vi "System Integrity Tool.vi"() -> ()   [LabVIEW 2010]
uses:
  SIT_Data.ctl
  Re-use Library/VIE.Module.Queued Message Handler.enqueue.State.PolyChild.QueuedMessageHandler.vi
  Re-use Library/VIE.Module.Queued Message Handler.[enqueue].State.PolyChild.QueuedMessageHandler.vi
  <vilib>/Utility/config.llb/Read Key (String).vi
  Re-use Library/Remove Duplicates from 1D Array (Path)__ogtk.vi
  Re-use Library/VIE.Module.Queued Message Handler.QueuedMessageHandler.dqGOOPClass.lvlib
  <vilib>/Utility/config.llb/NI_LVConfig.lvlib
panel:
  out "Error Out":errorcluster
  in  "Exit":bool
  in  "Add Package Integrity File":bool
  in  "Delete Package Integrity File":bool
  in  "Package Integrity Files":i32(listbox)
  in  "System Integrity File Path":path
  in  "Save System Integrity File":bool
  in  "User Name":string
  in  "Purpose":string
  in  "Package Revision":string
  in  "Package ID":string
  in  "Package Integrity File Path":path
  in  "Undo":bool
  in  "Save Package Integrity File":bool
  in  "Remove Selected Files":bool
  in  "Add VI Hierarchy":bool
  in  "Recursive":bool
  in  "Add Directory":bool
  in  "Add File":bool
  out "Selection Log":string
  in  "File List":i32[](listbox)
  in  "error in (no error)":errorcluster
  out "error out":errorcluster
  out "CVT (out)":T1
  # "Use the CVT as a data bus for data that is\nto be accesed outside of the VI.  It can be\nused for data passed around  inside the state\nmachine too, and all local data can be selectively\npurged from the CVT in the \"system.Exit\" state."
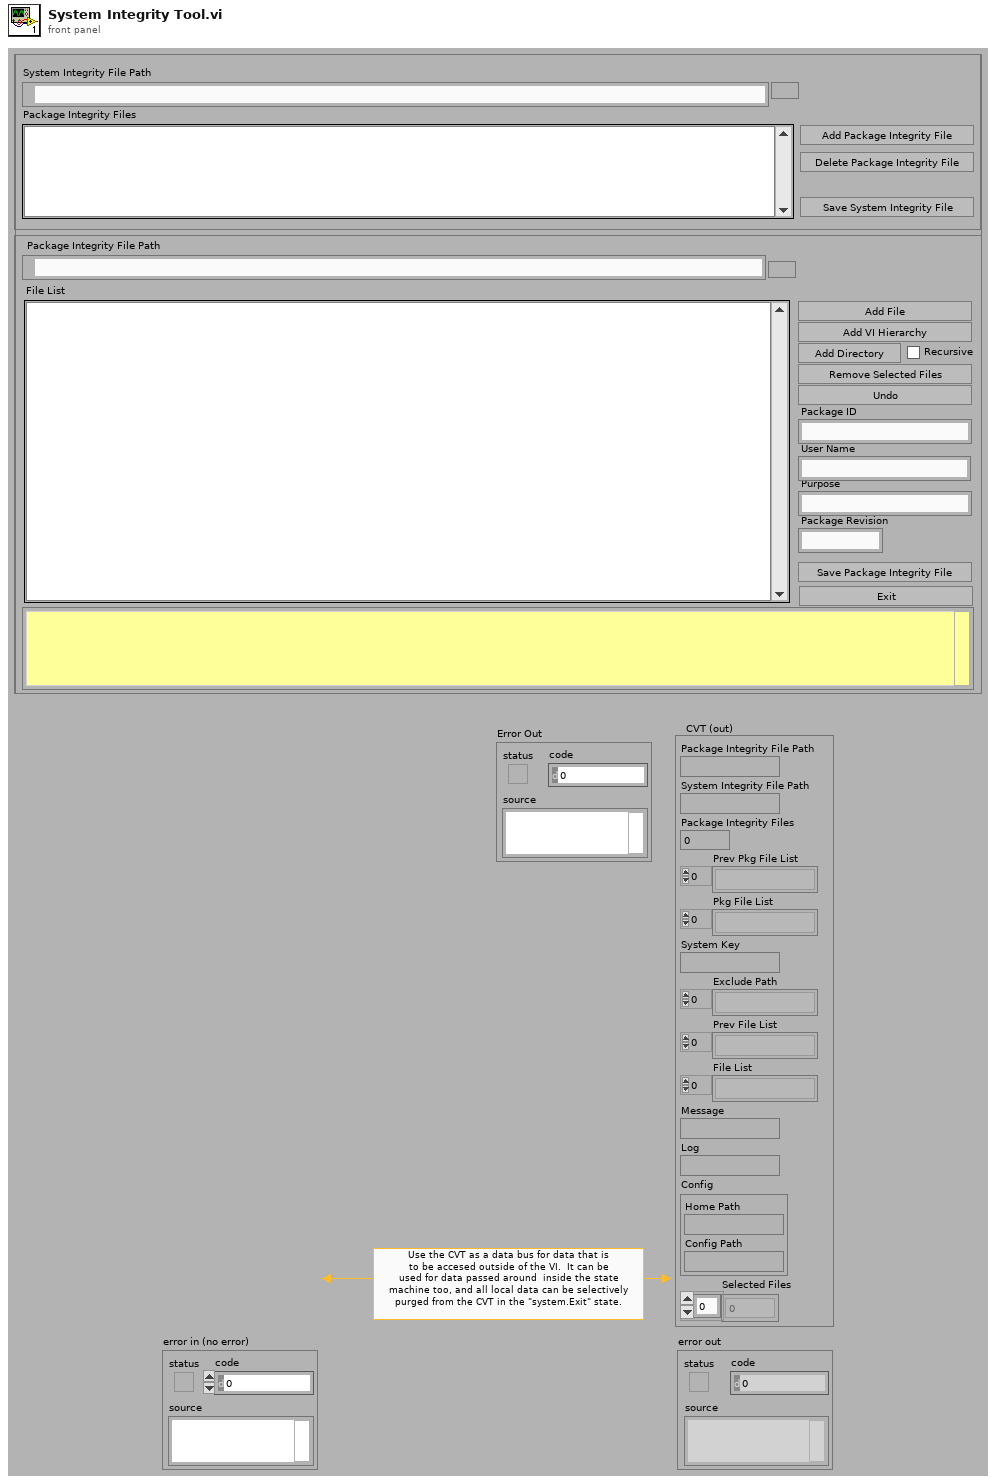
[diagram p1: front panel]
types:
  T1 = typedef "SIT_Data.ctl" = cluster{"Package Integrity File Path":path, "System Integrity File Path":path, "Package Integrity Files":i32, "Prev Pkg File List":path[], "Pkg File List":path[], "System Key":string, "Exclude Path":path[], "Prev File List":path[], "File List":path[], "Message":string, "Log":string, "Config":cluster{"Home Path":path, "Config Path":path}, "Selected Files":i32[]}
  T2 = typedef "VIE.Module.Queued Message Handler.QueuedMessageHandler.dqGOOPClass.lvlib/VIE.Module.Queued Message Handler.dqClass_ObjectReference.ctl" = refnum<k1>
  T3 = typedef "NI_LVConfig.lvlib/Config Data RefNum.ctl" = refnum<k1>
  T4 = enum32{"existing file", "new file", "new or existing file", "existing dir", "new dir", "new or existing dir", "existing file (use LLBs)", "new file (use LLBs)", "new or existing file (use LLBs)", "new or existing file or directory (use LLBs)", "existing dir (use LLBs)", "new dir (use LLBs)", "new or existing dir (use LLBs)", "existing file or dir", "new file or dir", "new or existing file or dir", "existing file or dir (use LLBs)", "new file or dir (use LLBs)"}
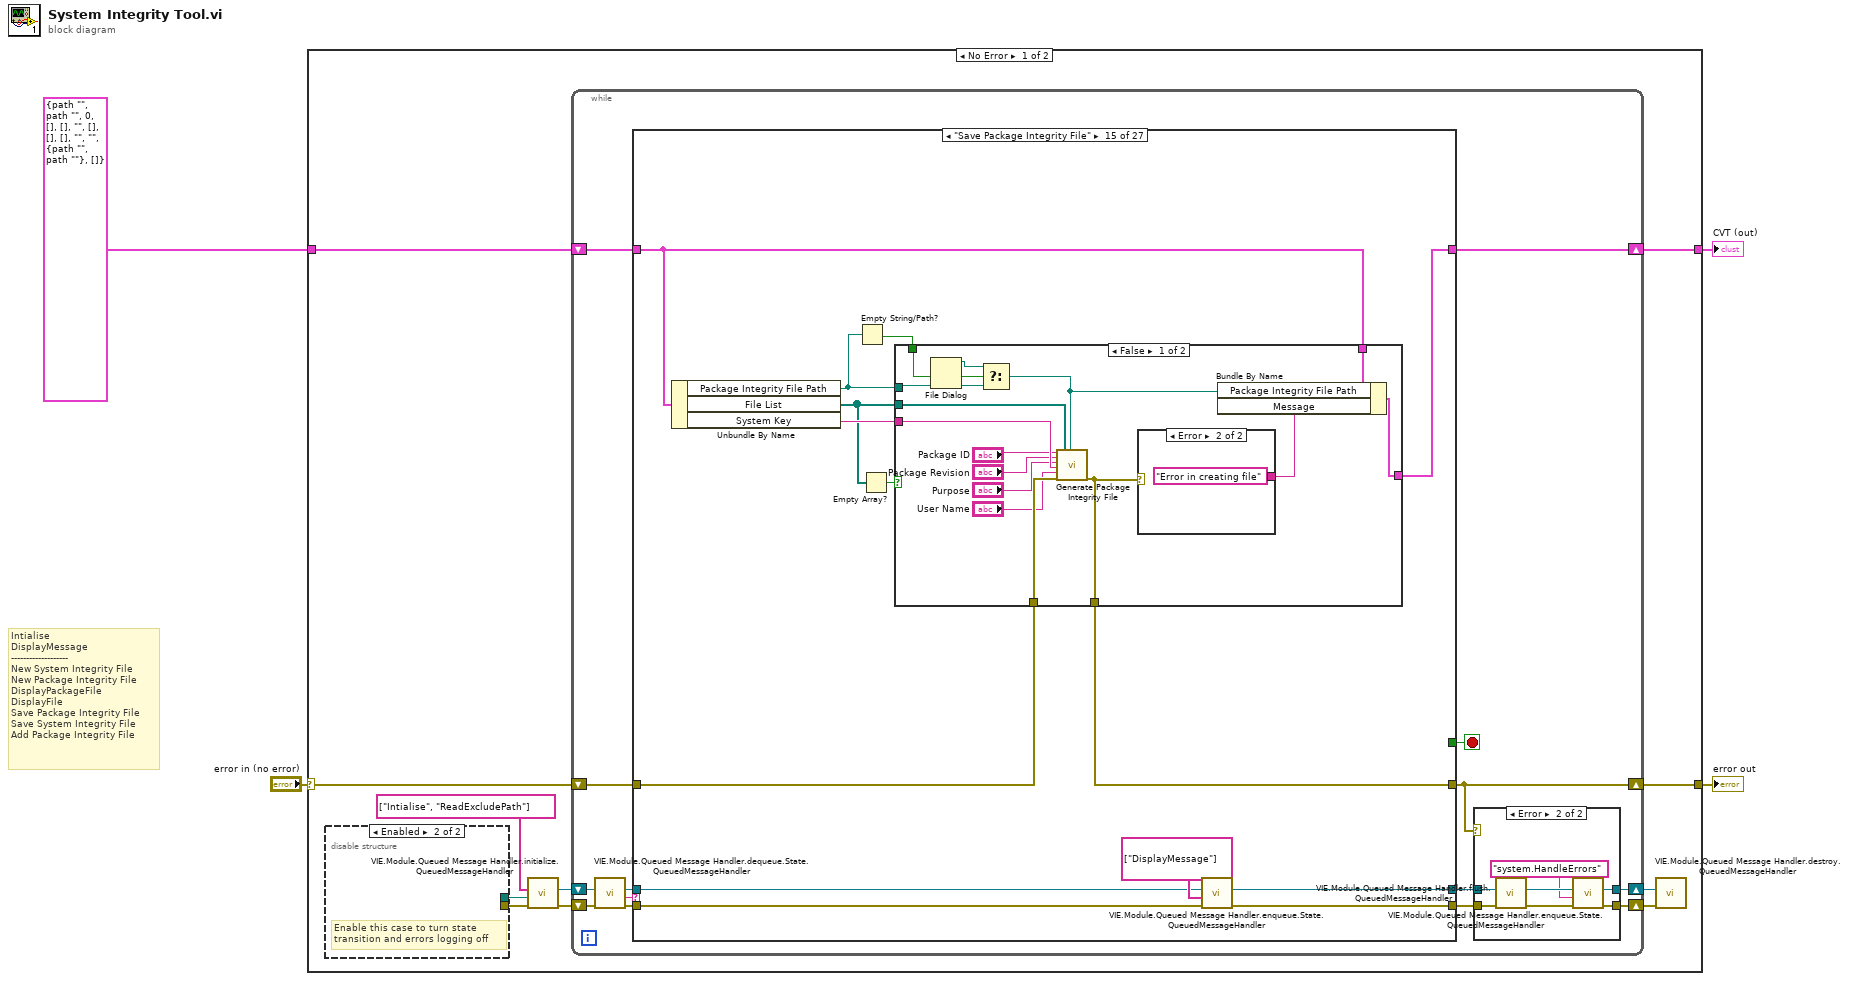
[diagram p0: block diagram]
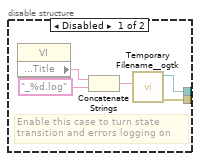
[diagram p2: hidden frame]
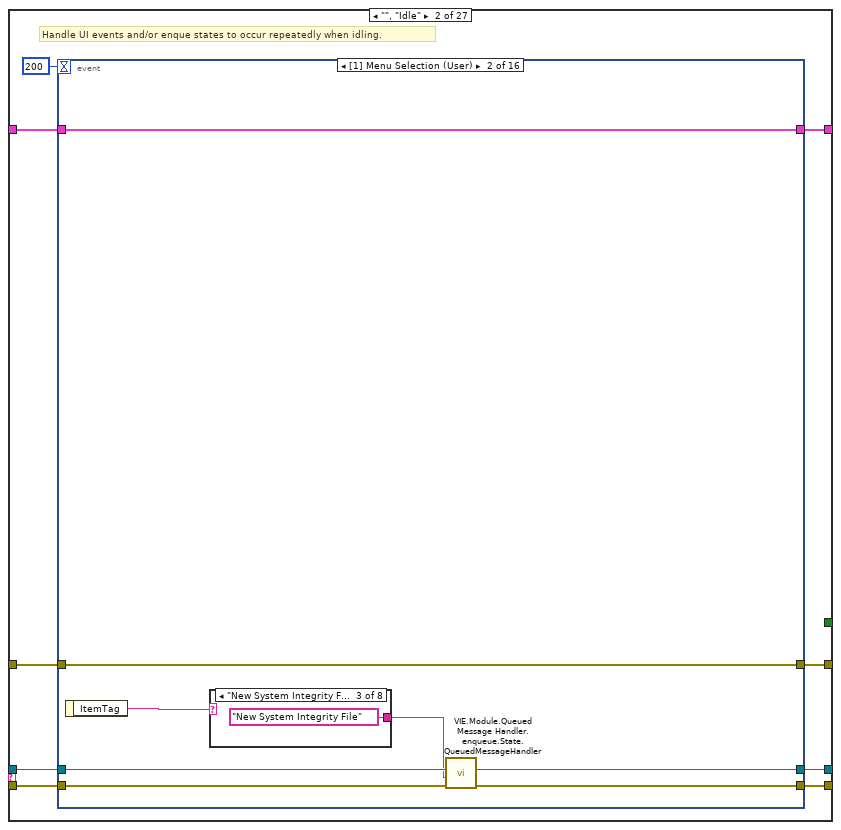
[diagram p5: hidden frame]
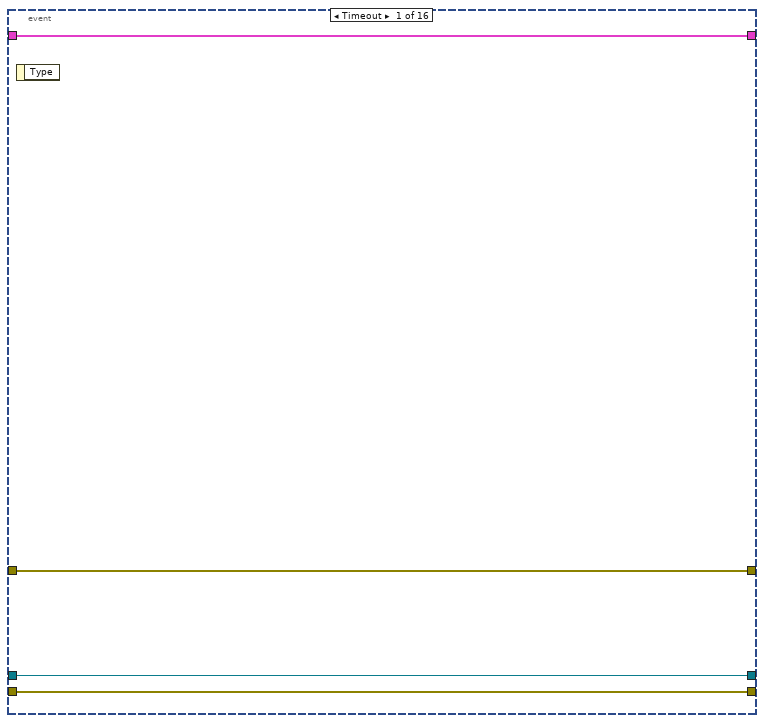
[diagram p6: hidden frame]
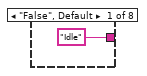
[diagram p7: hidden frame]
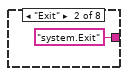
[diagram p8: hidden frame]
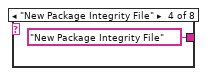
[diagram p9: hidden frame]
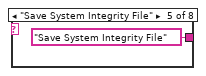
[diagram p10: hidden frame]
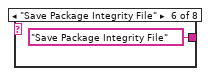
[diagram p11: hidden frame]
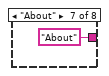
[diagram p12: hidden frame]
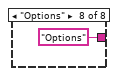
[diagram p13: hidden frame]
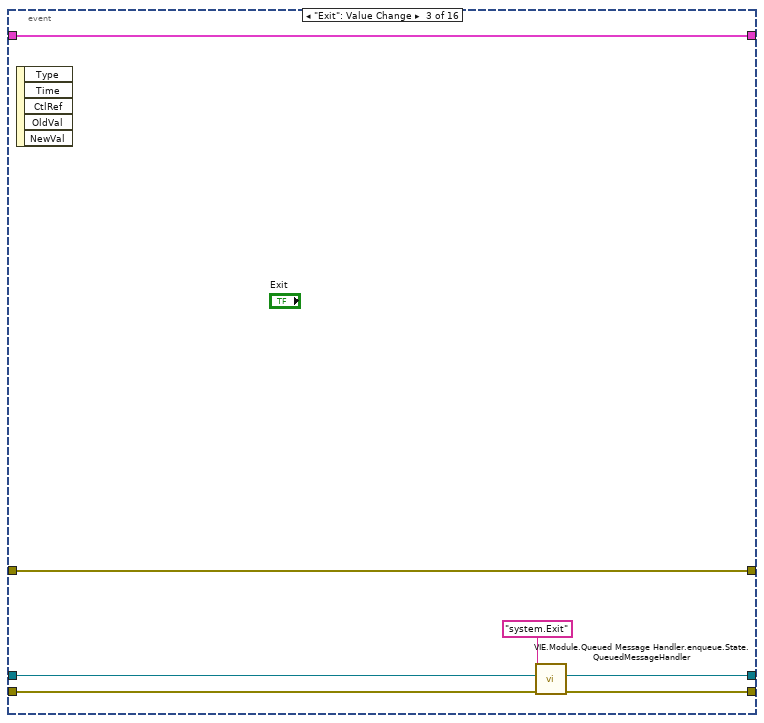
[diagram p14: hidden frame]
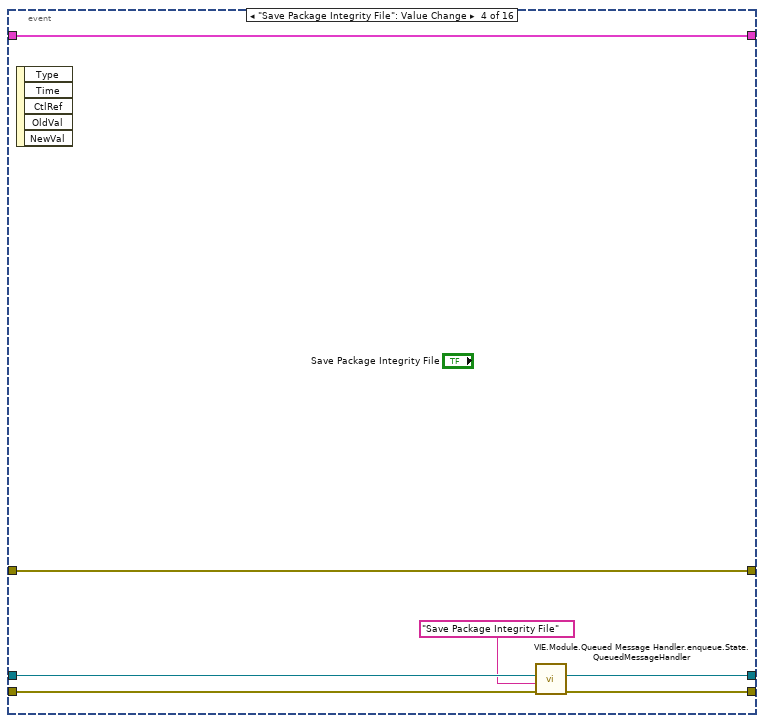
[diagram p15: hidden frame]
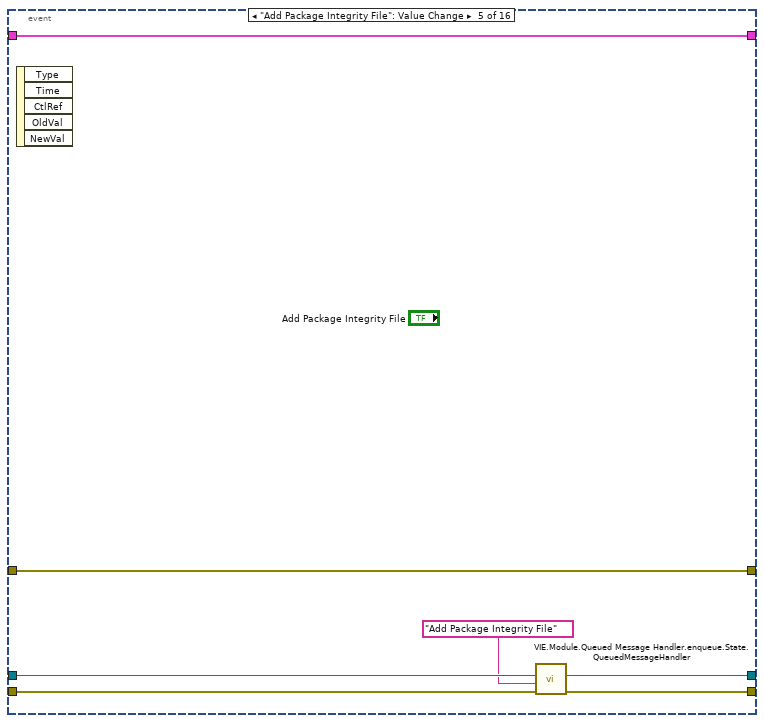
[diagram p16: hidden frame]
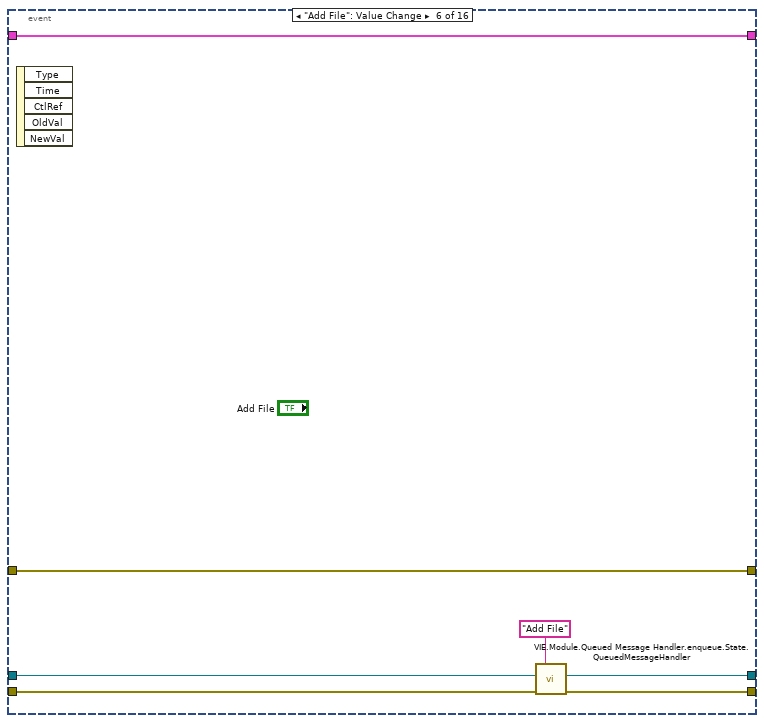
[diagram p17: hidden frame]
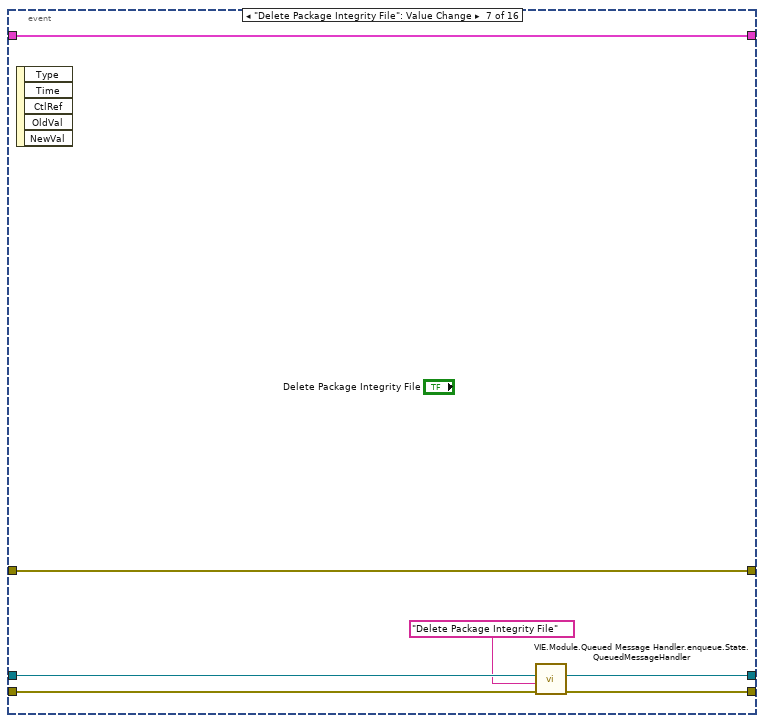
[diagram p18: hidden frame]
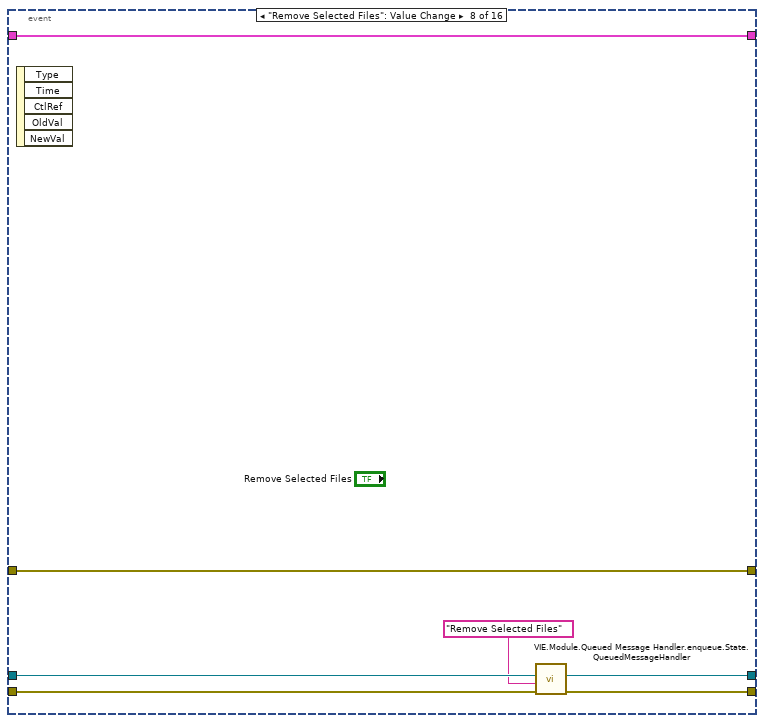
[diagram p19: hidden frame]
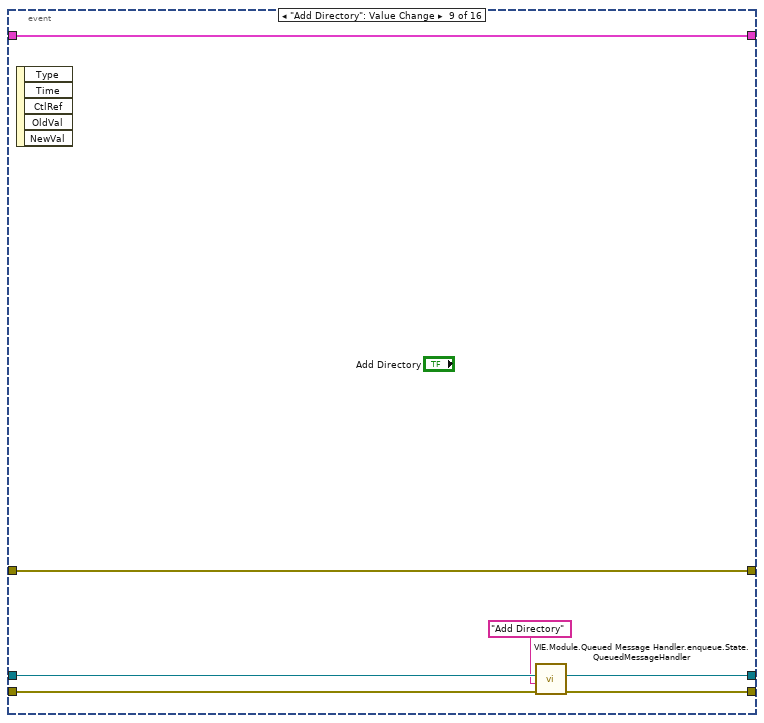
[diagram p20: hidden frame]
diagram:
  # "Intialise\nDisplayMessage\n-------------------\nNew System Integrity File\nNew Package Integrity File\nDisplayPackageFile\nDisplayFile\nSave Package Integrity File\nSave System Integrity File\nAdd Package Integrity File"
  n1 = case shown="No Error" "error in (no error)" {
    selector: "error in (no error)" -> [w8 w719]
    tunnel: [w7 w719] -> w2
    tunnel: T1 {"Package Integrity File Path"=path "", "System Integrity File Path"=path "", "Package Integrity Files"=0, "Prev Pkg File List"=[], "Pkg File List"=[], "System Key"="", "Exclude Path"=[], "Prev File List"=[], "File List"=[], "Message"="", "Log"="", "Config"={"Home Path"=path "", "Config Path"=path ""}, "Selected Files"=[]} ("CVT (in)") -> [w5 w718]
    tunnel: [w9 w718] -> w4
    frame No Error {
      n2 = disable-structure shown="Enabled" {
        disable-tunnel: [w17 _] -> w11
        disable-tunnel: [w16 _] -> w10
        frame Disabled {
          # "Enable this case to turn state\ntransition and errors logging on"
          n3 = property class="VI"() -> ("Front Panel.Title"=w18:string)  [unwired: 2 in, 2 out]
          n4 = Concatenate Strings(w18, "_%d.log" ("string")) -> (w20:string)
          n5 = call <userlib>:"Temporary Filename__ogtk.vi"("pattern (lvtemp%d.tmp)"=w20) -> ("error out"=w17:errorcluster, "file in tmp dir"=w16:path)  [unwired: 5 in]
        }
        frame Enabled {
          # "Enable this case to turn state\ntransition and errors logging off"
        }
      }
      n6 = call "VIE.Module.Queued Message Handler.initialize.QueuedMessageHandler.vi"("error in (no error)"=w11, "State Queue Log FilePath (\"\" = Do Not Log)"=w10, "Initial State Queue (empty)"=string[] ["Intialise", "ReadExcludePath"] ("Initial State Queue")) -> ("error out"=w15:errorcluster, "QueuedMessageHandler.dqGOOPClass (out)"=w12:T2)  [unwired: 7 in]
      n7 = while {
        shift-right: [w23] -> w14
        shift-left: w15 -> [w31]
        shift-right: [w28] -> w9
        shift-left: w5 -> [w29]
        shift-right: [w26] -> w7
        shift-left: w8 -> [w27]
        shift-right: [w22] -> w13
        shift-left: w12 -> [w34]
        stop <- w21 stop-if-true
        n8 = call "VIE.Module.Queued Message Handler.dequeue.State.QueuedMessageHandler.vi"("error in (no error)"=w31, "QueuedMessageHandler.dqGOOPClass (in)"=w34) -> ("error out"=w32:errorcluster, "State Dequeued"=w30:string, "QueuedMessageHandler.dqGOOPClass (out)"=w33:T2)  [unwired: 7 in]
        n9 = case shown="\"Save Package Integrity File\"" w30 {
          selector: w30 -> [_ _ _ _ _ _ _ _ _ _ _ _ _ _ _ _ _ _ _ _ _ _ _ _ w679 _ _]
          tunnel: w32 -> [w44 w54 w192 w199 w220 w225 w250 w256 w262 w278 w293 w334 w345 w373 w406 w442 w459 w492 w522 w555 w610 w625 w635 w673 w678 w696 w714]
          tunnel: [w44 w49 w189 w199 w220 w224 w248 w255 w262 w276 w291 w332 w344 w372 w405 w441 w458 w491 w521 w554 w609 w624 w634 w673 w678 w687 w714] -> w25
          tunnel: w33 -> [w45 w53 w191 w200 w221 w223 w251 w254 w263 w279 w294 w335 w343 w371 w404 w440 w457 w490 w520 w553 w608 w623 w633 w674 w677 w697 w715]
          tunnel: [w45 w50 w190 w200 w221 w222 w249 w253 w263 w277 w292 w333 w342 w370 w403 w439 w456 w489 w519 w552 w607 w622 w632 w674 w677 w688 w715] -> w24
          tunnel: w29 -> [w47 w56 w196 w202 w211 w234 w252 w259 w265 w272 w285 w324 w351 w376 w401 w433 w451 w484 w516 w549 w606 w621 w639 w676 w686 w700 w713]
          tunnel: [w47 w52 w195 w206 w210 w233 w252 w259 w265 w271 w289 w323 w350 w375 w400 w432 w450 w483 w515 w548 w605 w620 w638 w676 w686 w700 w713] -> w28
          tunnel: w27 -> [w46 w55 w197 w201 w219 w235 w246 w260 w264 w274 w287 w330 w356 w384 w399 _ w449 w482 w514 w547 w604 w619 w654 w675 w681 w698 w716]
          tunnel: [w46 w51 w183 w203 w219 w235 w246 w260 w264 w274 w286 w330 w356 w384 w398 w429 w448 w481 w513 w546 w604 w619 w654 w675 w680 w691 w716] -> w26
          tunnel: [_ _ _ _ _ _ _ _ _ _ _ _ _ _ _ _ _ _ _ _ _ _ _ _ _ _ TRUE] -> w21
          frame "---- Custom States --------------------------" {
            # "Do not put any code in here - this is a case divider, and is not a valid state, so any code here will not be executed."
          }
          frame "", "Idle" {
            # "Handle UI events and/or enque states to occur repeatedly when idling."
            n10 = event shown="[1] Menu Selection (User)" {
              selector: _ -> [_ _ _ _ _ _ _ _ _ _ _ _ _ _ _ _]
              dyn-events: _ -> [_ _ _ _ _ _ _ _ _ _ _ _ _ _ _ _]
              timeout: 200 -> [_ _ _ _ _ _ _ _ _ _ _ _ _ _ _ _]
              tunnel: w56 -> [w60 w68 w83 w90 w97 w104 w111 w118 w125 w132 w139 w146 w149 w159 w168 w179]
              tunnel: w55 -> [w57 w67 w82 w89 w96 w103 w110 w117 w124 w131 w138 w145 w155 w166 w175 w181]
              tunnel: w54 -> [w58 w66 w81 w88 w95 w102 w109 w116 w123 w130 w137 w144 w154 w165 w174 w176]
              tunnel: w53 -> [w59 w64 w79 w86 w93 w100 w107 w114 w121 w128 w135 w142 w152 w163 w172 w177]
              tunnel: [w60 w68 w83 w90 w97 w104 w111 w118 w125 w132 w139 w146 w148 w160 w169 w180] -> w52
              tunnel: [w57 w67 w82 w89 w96 w103 w110 w117 w124 w131 w138 w145 w155 w166 w175 w181] -> w51
              tunnel: [w59 w63 w78 w85 w92 w99 w106 w113 w120 w127 w134 w141 w151 w162 w171 w177] -> w50
              tunnel: [w58 w65 w80 w87 w94 w101 w108 w115 w122 w129 w136 w143 w153 w164 w173 w176] -> w49
              event Timeout {
                n11 = event-data() -> ()  [unwired: 1 in, 1 out]
              }
              event Menu Selection (User) {
                n12 = event-data() -> ("ItemTag"=w62:string)  [unwired: 1 in]
                n13 = case shown="\"New System Integrity File\"" w62 {
                  tunnel: ["Idle" ("ItemTag") "system.Exit" ("ItemTag") "New System Integrity File" ("ItemTag") "New Package Integrity File" ("ItemTag") "Save System Integrity File" ("ItemTag") "Save Package Integrity File" ("ItemTag") "About" ("ItemTag") "Options" ("ItemTag")] -> w61
                  frame "False", Default {
                  }
                  frame "Exit" {
                  }
                  frame "New System Integrity File" {
                  }
                  frame "New Package Integrity File" {
                  }
                  frame "Save System Integrity File" {
                  }
                  frame "Save Package Integrity File" {
                  }
                  frame "About" {
                  }
                  frame "Options" {
                  }
                }
                n14 = call-poly "VIE.Module.Queued Message Handler.enqueue.State.QueuedMessageHandler.vi"("error in (no error)"=w66, "State to Enqueue"=w61, "QueuedMessageHandler.dqGOOPClass (in)"=w64) -> ("error out"=w65:errorcluster, "QueuedMessageHandler.dqGOOPClass (out)"=w63:T2)  [unwired: 7 in]
              }
              event "Exit": Value Change {
                n15 = event-data() -> ()  [unwired: 1 in, 5 out]
                n16 = call-poly "VIE.Module.Queued Message Handler.enqueue.State.QueuedMessageHandler.vi"("error in (no error)"=w81, "State to Enqueue"="system.Exit", "QueuedMessageHandler.dqGOOPClass (in)"=w79) -> ("error out"=w80:errorcluster, "QueuedMessageHandler.dqGOOPClass (out)"=w78:T2)  [unwired: 7 in]
              }
              event "Save Package Integrity File": Value Change {
                n17 = event-data() -> ()  [unwired: 1 in, 5 out]
                n18 = call-poly "VIE.Module.Queued Message Handler.enqueue.State.QueuedMessageHandler.vi"("error in (no error)"=w88, "State to Enqueue"="Save Package Integrity File", "QueuedMessageHandler.dqGOOPClass (in)"=w86) -> ("error out"=w87:errorcluster, "QueuedMessageHandler.dqGOOPClass (out)"=w85:T2)  [unwired: 7 in]
              }
              event "Add Package Integrity File": Value Change {
                n19 = event-data() -> ()  [unwired: 1 in, 5 out]
                n20 = call-poly "VIE.Module.Queued Message Handler.enqueue.State.QueuedMessageHandler.vi"("error in (no error)"=w95, "State to Enqueue"="Add Package Integrity File", "QueuedMessageHandler.dqGOOPClass (in)"=w93) -> ("error out"=w94:errorcluster, "QueuedMessageHandler.dqGOOPClass (out)"=w92:T2)  [unwired: 7 in]
              }
              event "Add File": Value Change {
                n21 = event-data() -> ()  [unwired: 1 in, 5 out]
                n22 = call-poly "VIE.Module.Queued Message Handler.enqueue.State.QueuedMessageHandler.vi"("error in (no error)"=w102, "State to Enqueue"="Add File", "QueuedMessageHandler.dqGOOPClass (in)"=w100) -> ("error out"=w101:errorcluster, "QueuedMessageHandler.dqGOOPClass (out)"=w99:T2)  [unwired: 7 in]
              }
              event "Delete Package Integrity File": Value Change {
                n23 = event-data() -> ()  [unwired: 1 in, 5 out]
                n24 = call-poly "VIE.Module.Queued Message Handler.enqueue.State.QueuedMessageHandler.vi"("error in (no error)"=w109, "State to Enqueue"="Delete Package Integrity File", "QueuedMessageHandler.dqGOOPClass (in)"=w107) -> ("error out"=w108:errorcluster, "QueuedMessageHandler.dqGOOPClass (out)"=w106:T2)  [unwired: 7 in]
              }
              event "Remove Selected Files": Value Change {
                n25 = event-data() -> ()  [unwired: 1 in, 5 out]
                n26 = call-poly "VIE.Module.Queued Message Handler.enqueue.State.QueuedMessageHandler.vi"("error in (no error)"=w116, "State to Enqueue"="Remove Selected Files", "QueuedMessageHandler.dqGOOPClass (in)"=w114) -> ("error out"=w115:errorcluster, "QueuedMessageHandler.dqGOOPClass (out)"=w113:T2)  [unwired: 7 in]
              }
              event "Add Directory": Value Change {
                n27 = event-data() -> ()  [unwired: 1 in, 5 out]
                n28 = call-poly "VIE.Module.Queued Message Handler.enqueue.State.QueuedMessageHandler.vi"("error in (no error)"=w123, "State to Enqueue"="Add Directory", "QueuedMessageHandler.dqGOOPClass (in)"=w121) -> ("error out"=w122:errorcluster, "QueuedMessageHandler.dqGOOPClass (out)"=w120:T2)  [unwired: 7 in]
              }
              event "Add VI Hierarchy": Value Change {
                n29 = event-data() -> ()  [unwired: 1 in, 5 out]
                n30 = call-poly "VIE.Module.Queued Message Handler.enqueue.State.QueuedMessageHandler.vi"("error in (no error)"=w130, "State to Enqueue"="Add VI Hierarchy", "QueuedMessageHandler.dqGOOPClass (in)"=w128) -> ("error out"=w129:errorcluster, "QueuedMessageHandler.dqGOOPClass (out)"=w127:T2)  [unwired: 7 in]
              }
              event "Undo": Value Change {
                n31 = event-data() -> ()  [unwired: 1 in, 5 out]
                n32 = call-poly "VIE.Module.Queued Message Handler.enqueue.State.QueuedMessageHandler.vi"("error in (no error)"=w137, "State to Enqueue"="Undo", "QueuedMessageHandler.dqGOOPClass (in)"=w135) -> ("error out"=w136:errorcluster, "QueuedMessageHandler.dqGOOPClass (out)"=w134:T2)  [unwired: 7 in]
              }
              event "Save System Integrity File": Value Change {
                n33 = event-data() -> ()  [unwired: 1 in, 5 out]
                n34 = call-poly "VIE.Module.Queued Message Handler.enqueue.State.QueuedMessageHandler.vi"("error in (no error)"=w144, "State to Enqueue"="Save System Integrity File", "QueuedMessageHandler.dqGOOPClass (in)"=w142) -> ("error out"=w143:errorcluster, "QueuedMessageHandler.dqGOOPClass (out)"=w141:T2)  [unwired: 7 in]
              }
              event "System Integrity File Path": Value Change {
                n35 = event-data() -> ("NewVal"=w147:path)  [unwired: 1 in]
                n36 = Bundle By Name(cluster=w149, "System Integrity File Path"=w147) -> (w148:T1)
                n37 = call-poly "VIE.Module.Queued Message Handler.enqueue.State.QueuedMessageHandler.vi"("error in (no error)"=w154, "State to Enqueue"="Load System Integrity File", "QueuedMessageHandler.dqGOOPClass (in)"=w152) -> ("error out"=w153:errorcluster, "QueuedMessageHandler.dqGOOPClass (out)"=w151:T2)  [unwired: 7 in]
              }
              event "Package Integrity Files": Value Change {
                n38 = event-data() -> ("NewVal"=w156:i32)  [unwired: 1 in]
                n39 = Unbundle By Name(w159) -> ("Pkg File List"=w158:path[])
                n40 = Index Array(array=w158, index=w156) -> (element=w157:path)
                n41 = local write "Package Integrity File Path"(w157) -> ()
                n42 = Bundle By Name(cluster=w159, "Package Integrity File Path"=w157, "Package Integrity Files"=w156) -> (w160:T1)
                n43 = call-poly "VIE.Module.Queued Message Handler.enqueue.State.QueuedMessageHandler.vi"("error in (no error)"=w165, "State to Enqueue"="Load Package Integrity File", "QueuedMessageHandler.dqGOOPClass (in)"=w163) -> ("error out"=w164:errorcluster, "QueuedMessageHandler.dqGOOPClass (out)"=w162:T2)  [unwired: 7 in]
              }
              event "Package Integrity File Path": Value Change {
                n44 = event-data() -> ()  [unwired: 1 in, 1 out]
                n45 = Bundle By Name(cluster=w168, "Package Integrity File Path"="Package Integrity File Path") -> (w169:T1)
                n46 = call-poly "VIE.Module.Queued Message Handler.enqueue.State.QueuedMessageHandler.vi"("error in (no error)"=w174, "State to Enqueue"="Load Package Integrity File", "QueuedMessageHandler.dqGOOPClass (in)"=w172) -> ("error out"=w173:errorcluster, "QueuedMessageHandler.dqGOOPClass (out)"=w171:T2)  [unwired: 7 in]
              }
              event "File List": Value Change {
                n47 = event-data() -> ("NewVal"=w178:i32[])  [unwired: 1 in]
                n48 = Bundle By Name(cluster=w179, "Selected Files"=w178) -> (w180:T1)
              }
            }
          }
          frame "Intialise" {
            w184 = path "" ("Package Integrity File Path")
            w185 = string[] [] ("Item Names")
            n49 = call "Fit VI window to Largest Dec__ogtk.vi"("error in (no error)"=w197) -> ("error out"=w183:errorcluster)  [unwired: 5 in, 1 out]
            n50 = Current VI's Path() -> (path=w187:path)
            n51 = Strip Path(path=w187) -> (stripped path=w186:path)  [unwired: 1 out]
            n52 = Build Path(base path=w186, name or relative path="System Integrity Tool setting.ini") -> (appended path=w182:path)
            n53 = local write "System Integrity File Path"(w184) -> ()
            n54 = local write "Package Integrity File Path"(w184) -> ()
            n55 = Bundle By Name(cluster=w196, "Message"="Welcome to the Package Integrity File Generation Utility, brought to you by VI Engineering, Inc." ("queue element"), "Config.Home Path"=w186, "Config.Config Path"=w182) -> (w195:T1)
            n56 = property on="Package Integrity Files" class="LstBox (strict)"("Item Names"=w185) -> ()  [unwired: 2 in, 2 out]
            n57 = property on="File List" class="LstBox (strict)"("Item Names"=w185) -> ()  [unwired: 2 in, 2 out]
            n58 = call-poly "VIE.Module.Queued Message Handler.enqueue.State.QueuedMessageHandler.vi"("error in (no error)"=w192, "State to Enqueue"="DisplayMessage", "QueuedMessageHandler.dqGOOPClass (in)"=w191) -> ("error out"=w189:errorcluster, "QueuedMessageHandler.dqGOOPClass (out)"=w190:T2)  [unwired: 7 in]
          }
          frame "ReadExcludePath" {
            n59 = Unbundle By Name(w202) -> ("Config.Config Path"=w198:path)
            n60 = call "Read Write Exclude path.vi"("path In"=w198, "Error In"=w201) -> ("Key out"=w205:string, "Exclude Path Out"=w204:path[], "Error Out"=w203:errorcluster)  [unwired: 10 in, 1 out]
            n61 = Bundle By Name(cluster=w202, "System Key"=w205, "Exclude Path"=w204) -> (w206:T1)
          }
          frame "DisplayMessage" {
            n62 = Unbundle By Name(w211) -> ("Log"=w214:string, "Message"=w208:string)
            n63 = Empty String/Path?(string/path=w208) -> (empty?=w218:bool)
            n64 = Select(t="", s=w218, f="\r") -> (s? t:f=w216:string)
            n65 = Concatenate Strings(w214, w216, w208) -> (w213:string)
            n66 = call "SIT_Limit Display.vi"("Limit"=100 ("Number of Lines"), "Data In"=w213) -> ("Line Count"=w207:i32, "Data Out"=w209:string)  [unwired: 8 in]
            "Selection Log" <- w209
            n67 = property on="Selection Log" class="Str"("Text.Scroll Position"=w207) -> ()  [unwired: 2 in, 2 out]
            n68 = Bundle By Name(cluster=w211, "Log"=w209) -> (w210:T1)
          }
          frame "Undo" {
            n69 = Unbundle By Name(w234) -> ("Prev File List"=w228:path[], "File List"=w227:path[])
            n70 = Array Size(array=w228) -> (size(s)=w231:i32)
            n71 = Array Size(array=w227) -> (size(s)=w230:i32)
            n72 = Greater?(x=w231, y=w230) -> (0:w232:bool)
            n73 = case shown="True" w232 {
              tunnel: w231 -> [w238 w244]
              tunnel: w230 -> [w237 w243]
              tunnel: [w236 w241] -> w229
              frame False {
                n74 = Subtract(x=w237, y=w238) -> (x-y=w240:i32)
                n75 = Format Into String(format string="Undo: %d File(s) Removed from List" ("Format String"), w240) -> (resulting string=w236:string)  [unwired: 2 in, 1 out]
              }
              frame True {
                n76 = Subtract(x=w244, y=w243) -> (x-y=w242:i32)
                n77 = Format Into String(format string="Undo: %d File(s) Added Back to List" ("Format String"), w242) -> (resulting string=w241:string)  [unwired: 2 in, 1 out]
              }
            }
            n78 = call-poly "VIE.Module.Queued Message Handler.enqueue.State.QueuedMessageHandler.vi"("error in (no error)"=w225, "States to Enqueue"=string[] ["DisplayMessage", "DisplayFile"], "QueuedMessageHandler.dqGOOPClass (in)"=w223) -> ("error out"=w224:errorcluster, "QueuedMessageHandler.dqGOOPClass (out)"=w222:T2)  [unwired: 7 in]
            n79 = Bundle By Name(cluster=w234, "File List"=w228, "Prev File List"=w227, "Message"=w229) -> (w233:T1)
          }
          frame "custom.CleanUp" {
            n80 = call-poly "VIE.Module.Queued Message Handler.enqueue.State.QueuedMessageHandler.vi"("error in (no error)"=w250, "State to Enqueue"="system.Exit", "QueuedMessageHandler.dqGOOPClass (in)"=w251) -> ("error out"=w248:errorcluster, "QueuedMessageHandler.dqGOOPClass (out)"=w249:T2)  [unwired: 7 in]
          }
          frame "Options" {
            n81 = Unbundle By Name(w259) -> ("Config.Config Path"=w258:path)
            n82 = call "Exclude Path Options.vi"("Error In"=w260, "Path In"=w258) -> ()  [unwired: 9 in, 1 out]
            n83 = call-poly "VIE.Module.Queued Message Handler.enqueue.State.QueuedMessageHandler.vi"("error in (no error)"=w256, "State to Enqueue"="ReadExcludePath", "QueuedMessageHandler.dqGOOPClass (in)"=w254) -> ("error out"=w255:errorcluster, "QueuedMessageHandler.dqGOOPClass (out)"=w253:T2)  [unwired: 7 in]
          }
          frame "About" {
            n84 = One Button Dialog(message="Purpose of this tool is for System Integrity") -> ()  [unwired: 1 in, 1 out]
          }
          frame "Load Package Integrity File" {
            n85 = Unbundle By Name(w272) -> ("Package Integrity File Path"=w273:path)
            n86 = call "Load Package Config.vi"("Path"=w273) -> ("Path Out"=w270:path[], "Package ID"=w269:string, "Purpose"=w268:string, "Package Revision"=w267:string, "Error Out"=→"Error Out":errorcluster)  [unwired: 9 in, 1 out]
            n87 = local write "Purpose"(w268) -> ()
            n88 = local write "Package Revision"(w267) -> ()
            n89 = local write "Package ID"(w269) -> ()
            n90 = call-poly "VIE.Module.Queued Message Handler.enqueue.State.QueuedMessageHandler.vi"("error in (no error)"=w278, "State to Enqueue"="DisplayFile", "QueuedMessageHandler.dqGOOPClass (in)"=w279) -> ("error out"=w276:errorcluster, "QueuedMessageHandler.dqGOOPClass (out)"=w277:T2)  [unwired: 7 in]
            n91 = Bundle By Name(cluster=w272, "Prev File List"=w270, "File List"=w270) -> (w271:T1)
          }
          frame "Load System Integrity File" {
            n92 = Unbundle By Name(w285) -> ("System Integrity File Path"=w284:path)
            n93 = call <vilib>:"Open Config Data.vi"("error in (no error)"=w287, "create file if necessary (T)"=FALSE, "configuration file path"=w284) -> ("error out"=w280:errorcluster, "refnum"=w288:T3)  [unwired: 6 in, 1 out]
            n94 = case shown="No Error" w280 {
              selector: w280 -> [w295 _]
              tunnel: w288 -> [w300 _]
              tunnel: [w299 _] -> w286
              tunnel: [w298 _] -> w283
              frame No Error {
                w306 = "Package Integrity Files" ("section")
                n95 = call <vilib>:"Get Key Names.vi"("section"=w306, "error in (no error)"=w295, "refnum"=w300) -> ("error out"=w305:errorcluster, "key names"=w307:string[], "refnum out"=w304:T3)  [unwired: 5 in, 1 out]
                n96 = for {
                  tunnel: w307 -> [w316] mode=indexing
                  tunnel: w306 -> [w315]
                  tunnel: w305 -> [w314]
                  tunnel: [w313] -> w303
                  tunnel: w304 -> [w312]
                  tunnel: [w311] -> w302
                  tunnel: [w309] -> w301 mode=indexing
                  n97 = call-poly <vilib>:"Read Key.vi"("section"=w315, "error in (no error)"=w314, "default value"="", "key"=w316, "refnum"=w312) -> ("error out"=w313:errorcluster, "value"=w309:string, "refnum out"=w311:T3)  [unwired: 3 in, 1 out]
                }
                n98 = call <vilib>:"Close Config Data.vi"("error in (no error)"=w303, "write file if changed (T)"=FALSE, "refnum"=w302) -> ("error out"=w299:errorcluster, "file path"=w297:path)  [unwired: 7 in]
                n99 = Strip Path(path=w297) -> (stripped path=w296:path)  [unwired: 1 out]
                n100 = for "Extract File Paths" {
                  tunnel: w301 -> [w320] mode=indexing
                  tunnel: [w318] -> w298 mode=indexing
                  tunnel: w296 -> [w317]
                  n101 = String To Path(string=w320) -> (path=w319:path)
                  n102 = call "Rel to Abs Path.vi"("Rel File Path"=w319, "Base Path"=w317) -> ("Path Out"=w318:path)  [unwired: 8 in, 1 out]
                }
              }
              frame Error {
              }
            }
            n103 = call-poly "VIE.Module.Queued Message Handler.enqueue.State.QueuedMessageHandler.vi"("error in (no error)"=w293, "State to Enqueue"="DisplayFile", "QueuedMessageHandler.dqGOOPClass (in)"=w294) -> ("error out"=w291:errorcluster, "QueuedMessageHandler.dqGOOPClass (out)"=w292:T2)  [unwired: 7 in]
            n104 = Index Array(array=w283) -> (element=w282:path)  [unwired: 1 in]
            n105 = Bundle By Name(cluster=w285, "Prev Pkg File List"=w283, "Pkg File List"=w283, "Package Integrity File Path"=w282) -> (w289:T1)
          }
          frame "New System Integrity File" {
            (unwired) T4."new file" ("select mode (2)")
            n106 = Unbundle By Name(w324) -> ("System Integrity File Path"=w325:path)
            n107 = Strip Path(path=w325) -> (stripped path=w329:path)  [unwired: 1 out]
            n108 = File Dialog(6:"*.vsi" ("pattern"), 7:"New System Integrity File" ("prompt"), 11:w329) -> (0:w326:errorcluster, 1:w321:bool, 3:w322:path)  [unwired: 4 in, 1 out]
            n109 = case shown="False" w321 {
              tunnel: w326 -> [_ _]
              tunnel: w324 -> [w340 w341]
              tunnel: [w339 w341] -> w323
              tunnel: w322 -> [w337 _]
              frame False {
                w338 = path[] []
                n110 = Bundle By Name(cluster=w340, "Prev Pkg File List"=w338, "Pkg File List"=w338, "System Integrity File Path"=w337) -> (w339:T1)
                n111 = property on="Package Integrity Files" class="LstBox (strict)"("Value"=-1 ("Package Integrity Files")) -> ()  [unwired: 2 in, 2 out]
                n112 = local write "System Integrity File Path"(w337) -> ()
              }
              frame True {
              }
            }
            n113 = call-poly "VIE.Module.Queued Message Handler.enqueue.State.QueuedMessageHandler.vi"("error in (no error)"=w334, "State to Enqueue"="DisplayPackageFile", "QueuedMessageHandler.dqGOOPClass (in)"=w335) -> ("error out"=w332:errorcluster, "QueuedMessageHandler.dqGOOPClass (out)"=w333:T2)  [unwired: 7 in]
          }
          frame "New Package Integrity File" {
            n114 = Unbundle By Name(w351) -> ("System Integrity File Path"=w352:path)
            n115 = Strip Path(path=w352) -> (stripped path=w355:path)  [unwired: 1 out]
            n116 = File Dialog(6:"*.vpi" ("pattern"), 7:"New Package Integrity File" ("prompt"), 11:w355) -> (0:w347:errorcluster, 1:w348:bool, 3:w349:path)  [unwired: 4 in, 1 out]
            n117 = case shown="False" w348 {
              tunnel: w351 -> [w360 w366]
              tunnel: [w359 w366] -> w350
              tunnel: w349 -> [w358 _]
              tunnel: w347 -> [_ _]
              frame False {
                w357 = path[] [] ("Prev File List")
                n118 = local write "Package Integrity File Path"(w358) -> ()
                n119 = Strip Path(path=w358) -> (name=w364:string)  [unwired: 1 out]
                n120 = Bundle By Name(cluster=w360, "File List"=w357, "Prev File List"=w357, "Package Integrity File Path"=w358) -> (w359:T1)
                n121 = property on="Package Integrity Files" class="LstBox (strict)"("Value"=-1 ("Package Integrity Files")) -> ()  [unwired: 2 in, 2 out]
                n122 = local write "Package Revision"("") -> ()
                n123 = Match Pattern(string=w364, regular expression=".vpi$") -> (before substring=w361:string)  [unwired: 1 in, 3 out]
                n124 = local write "Package ID"(w361) -> ()
              }
              frame True {
              }
            }
            n125 = call-poly "VIE.Module.Queued Message Handler.enqueue.State.QueuedMessageHandler.vi"("error in (no error)"=w345, "State to Enqueue"="DisplayFile", "QueuedMessageHandler.dqGOOPClass (in)"=w343) -> ("error out"=w344:errorcluster, "QueuedMessageHandler.dqGOOPClass (out)"=w342:T2)  [unwired: 7 in]
          }
          frame "DisplayPackageFile" {
            # "Message Queue"
            n126 = Unbundle By Name(w376) -> ("System Integrity File Path"=w377:path, "Pkg File List"=w369:path[])
            n127 = call-poly "Remove Duplicates from 1D Array__ogtk.vi"("Input Array"=w369) -> ("Output Array"=w383:path[])  [unwired: 1 out]
            n128 = Strip Path(path=w377) -> (stripped path=w378:path)  [unwired: 1 out]
            n129 = Sort 1D Array(array=w383) -> (sorted array=w367:path[])
            n130 = Array Size(array=w369) -> (size(s)=w381:i32)
            n131 = Array Size(array=w367) -> (size(s)=w380:i32)
            n132 = Not Equal?(x=w381, y=w380) -> (x != y?=w382:bool)
            n133 = case shown="True" w382 {
              tunnel: w381 -> [_ w392]
              tunnel: w380 -> [_ w393]
              tunnel: [_ w389] -> w368
              frame False {
              }
              frame True {
                n134 = Subtract(x=w392, y=w393) -> (x-y=w390:i32)
                n135 = Format Into String(format string="    %d Repeated File(s) Found and Removed from System Integrity File list" ("Format String"), w390) -> (resulting string=w389:string)  [unwired: 2 in, 1 out]
              }
            }
            n136 = for {
              tunnel: w378 -> [w388]
              tunnel: w367 -> [w387] mode=indexing
              tunnel: [w385] -> w379 mode=indexing
              n137 = call "Abs to Rel Path.vi"("File Path"=w387, "Base Path"=w388) -> ("Path Out"=w386:path)  [unwired: 8 in, 1 out]
              n138 = Path To String(path=w386) -> (string=w385:string)
            }
            n139 = call-poly "VIE.Module.Queued Message Handler.enqueue.State.QueuedMessageHandler.vi"("error in (no error)"=w373, "States to Enqueue"=string[] ["DisplayMessage"], "QueuedMessageHandler.dqGOOPClass (in)"=w371) -> ("error out"=w372:errorcluster, "QueuedMessageHandler.dqGOOPClass (out)"=w370:T2)  [unwired: 7 in]
            n140 = property on="Package Integrity Files" class="LstBox (strict)"("Item Names"=w379) -> ()  [unwired: 2 in, 2 out]
            n141 = Bundle By Name(cluster=w376, "Pkg File List"=w367, "Message"=w368) -> (w375:T1)
          }
          frame "Save Package Integrity File" {
            n142 = Unbundle By Name(w401) -> ("Package Integrity File Path"=w397:path, "File List"=w396:path[], "System Key"=w402:string)
            n143 = Empty String/Path?(string/path=w397) -> (empty?=w394:bool)
            n144 = Empty Array?(array=w396) -> (empty?=w395:bool)
            n145 = case shown="False" w395 {
              tunnel: w402 -> [w422 _]
              tunnel: w401 -> [w421 w428]
              tunnel: [w420 w426] -> w400
              tunnel: w399 -> [w419 w427]
              tunnel: [w418 w427] -> w398
              tunnel: w397 -> [w409 _]
              tunnel: w396 -> [w417 _]
              tunnel: w394 -> [w411 _]
              frame False {
                n146 = File Dialog() -> (3:w410:path)  [unwired: 7 in, 3 out]
                n147 = Select(t=w410, s=w411, f=w409) -> (s? t:f=w408:path)
                n148 = call "Generate Package Integrity File.vi"("PackageID"="Package ID", "PackageRev"="Package Revision", "Purpose"="Purpose", "System Key"=w422, "USER_NAME"="User Name", "Error In"=w419, "Package File Paths"=w417, "Integrity File Path"=w408) -> ("error out"=w418:errorcluster)  [unwired: 11 in]
                n149 = case shown="Error" w418 {
                  tunnel: ["Create Package Integrity File...Done..." ("Message") "Error in creating file" ("Message")] -> w412
                  frame No Error {
                  }
                  frame Error {
                  }
                }
                n150 = Bundle By Name(cluster=w421, "Package Integrity File Path"=w408, "Message"=w412) -> (w420:T1)
              }
              frame True {
                n151 = Bundle By Name(cluster=w428, "Message"="") -> (w426:T1)
              }
            }
            n152 = call-poly "VIE.Module.Queued Message Handler.enqueue.State.QueuedMessageHandler.vi"("error in (no error)"=w406, "States to Enqueue"=string[] ["DisplayMessage"], "QueuedMessageHandler.dqGOOPClass (in)"=w404) -> ("error out"=w405:errorcluster, "QueuedMessageHandler.dqGOOPClass (out)"=w403:T2)  [unwired: 7 in]
          }
          frame "Save System Integrity File" {
            n153 = Unbundle By Name(w433) -> ("System Integrity File Path"=w438:path, "Pkg File List"=w437:path[], "System Key"=w436:string)
            n154 = local read "User Name"() -> (w435:string)
            n155 = call "Generate System Integrity File.vi"("System Integrity File Path"=w438, "File Paths"=w437, "System Key"=w436, "USER_NAME"=w435) -> ("Error Out"=w429:errorcluster)  [unwired: 15 in]
            n156 = case shown="Error" w429 {
              tunnel: ["Done..." ("Message") "There was an error creating the System Integrity File" ("queue element")] -> w430
              frame No Error {
              }
              frame Error {
              }
            }
            n157 = call-poly "VIE.Module.Queued Message Handler.enqueue.State.QueuedMessageHandler.vi"("error in (no error)"=w442, "States to Enqueue"=string[] ["DisplayMessage"], "QueuedMessageHandler.dqGOOPClass (in)"=w440) -> ("error out"=w441:errorcluster, "QueuedMessageHandler.dqGOOPClass (out)"=w439:T2)  [unwired: 7 in]
            n158 = Concatenate Strings("Create System Integrity File....." ("Message"), w430) -> (w431:string)
            n159 = Bundle By Name(cluster=w433, "Message"=w431) -> (w432:T1)
          }
          frame "Add File" {
            n160 = Unbundle By Name(w451) -> ("File List"=w446:path[], "Package Integrity File Path"=w454:path)
            n161 = Strip Path(path=w454) -> (stripped path=w455:path)  [unwired: 1 out]
            n162 = File Dialog(11:w455) -> (0:w452:errorcluster, 1:w453:bool, 3:w447:path)  [unwired: 6 in, 1 out]
            n163 = case shown="False" w453 {
              tunnel: w459 -> [w472 w475]
              tunnel: [w471 w475] -> w458
              tunnel: w457 -> [w470 w476]
              tunnel: [w469 w476] -> w456
              tunnel: w452 -> [_ _]
              tunnel: w451 -> [w468 w477]
              tunnel: [w467 w477] -> w450
              tunnel: [w466 w474] -> w448
              tunnel: w449 -> [w466 w474]
              tunnel: w447 -> [w464 _]
              tunnel: w446 -> [w465 _]
              frame False {
                n164 = Path To String(path=w464) -> (string=w462:string)
                n165 = Build Array (concatenate)(w465, w464) -> (w463:path[])
                n166 = Concatenate Strings("Added File: " ("Message"), w462) -> (w461:string)
                n167 = call-poly "VIE.Module.Queued Message Handler.enqueue.State.QueuedMessageHandler.vi"("error in (no error)"=w472, "States to Enqueue"=string[] ["DisplayMessage", "DisplayFile"], "QueuedMessageHandler.dqGOOPClass (in)"=w470) -> ("error out"=w471:errorcluster, "QueuedMessageHandler.dqGOOPClass (out)"=w469:T2)  [unwired: 7 in]
                n168 = Bundle By Name(cluster=w468, "Prev File List"=w465, "File List"=w463, "Message"=w461) -> (w467:T1)
              }
              frame True {
              }
            }
          }
          frame "Add Package Integrity File" {
            n169 = Unbundle By Name(w484) -> ("Pkg File List"=w479:path[], "System Integrity File Path"=w487:path)
            n170 = Strip Path(path=w487) -> (stripped path=w488:path)  [unwired: 1 out]
            n171 = File Dialog(6:"*.vpi" ("pattern (all files)"), 11:w488) -> (0:w485:errorcluster, 1:w486:bool, 3:w480:path)  [unwired: 5 in, 1 out]
            n172 = case shown="False" w486 {
              tunnel: w492 -> [w505 w508]
              tunnel: [w504 w508] -> w491
              tunnel: w490 -> [w503 w509]
              tunnel: [w502 w509] -> w489
              tunnel: w485 -> [_ _]
              tunnel: w484 -> [w501 w510]
              tunnel: [w500 w510] -> w483
              tunnel: [w499 w507] -> w481
              tunnel: w482 -> [w499 w507]
              tunnel: w480 -> [w497 _]
              tunnel: w479 -> [w498 _]
              frame False {
                n173 = Path To String(path=w497) -> (string=w495:string)
                n174 = Build Array (concatenate)(w498, w497) -> (w496:path[])
                n175 = Concatenate Strings("Added Package Integrity File: " ("Message"), w495) -> (w494:string)
                n176 = call-poly "VIE.Module.Queued Message Handler.enqueue.State.QueuedMessageHandler.vi"("error in (no error)"=w505, "States to Enqueue"=string[] ["DisplayMessage", "DisplayPackageFile"], "QueuedMessageHandler.dqGOOPClass (in)"=w503) -> ("error out"=w504:errorcluster, "QueuedMessageHandler.dqGOOPClass (out)"=w502:T2)  [unwired: 7 in]
                n177 = Bundle By Name(cluster=w501, "Prev Pkg File List"=w498, "Pkg File List"=w496, "Message"=w494) -> (w500:T1)
              }
              frame True {
              }
            }
          }
          frame "Add Directory" {
            n178 = Unbundle By Name(w516) -> ("File List"=w511:path[])
            n179 = File Dialog() -> (0:w517:errorcluster, 1:w518:bool, 3:w512:path)  [unwired: 7 in, 1 out]
            n180 = case shown="False" w518 {
              tunnel: w522 -> [w537 w540]
              tunnel: [w536 w540] -> w521
              tunnel: w520 -> [w535 w541]
              tunnel: [w534 w541] -> w519
              tunnel: w517 -> [_ _]
              tunnel: w516 -> [w533 w542]
              tunnel: [w532 w542] -> w515
              tunnel: [w531 w539] -> w513
              tunnel: w514 -> [w531 w539]
              tunnel: w512 -> [w528 _]
              tunnel: w511 -> [w530 _]
              frame False {
                n181 = call "Get Recursive File details.vi"("Recursive?"="Recursive", "Path"=w528) -> ("Count"=w525:i32, "File Details"=w527:path[])  [unwired: 8 in]
                n182 = Build Array (concatenate)(w530, w527) -> (w529:path[])
                n183 = Format Into String(format string="Added %d File: " ("Message"), w525) -> (resulting string=w523:string)  [unwired: 2 in, 1 out]
                n184 = call-poly "VIE.Module.Queued Message Handler.enqueue.State.QueuedMessageHandler.vi"("error in (no error)"=w537, "States to Enqueue"=string[] ["DisplayMessage", "DisplayFile"], "QueuedMessageHandler.dqGOOPClass (in)"=w535) -> ("error out"=w536:errorcluster, "QueuedMessageHandler.dqGOOPClass (out)"=w534:T2)  [unwired: 7 in]
                n185 = Bundle By Name(cluster=w533, "Prev File List"=w530, "File List"=w529, "Message"=w523) -> (w532:T1)
              }
              frame True {
              }
            }
          }
          frame "Add VI Hierarchy" {
            n186 = Unbundle By Name(w549) -> ("File List"=w544:path[])
            n187 = File Dialog(6:"*.vi" ("pattern")) -> (0:w550:errorcluster, 1:w551:bool, 3:w545:path)  [unwired: 6 in, 1 out]
            n188 = case shown="False" w551 {
              tunnel: w555 -> [w570 w593]
              tunnel: [w569 w593] -> w554
              tunnel: w553 -> [w568 w594]
              tunnel: [w567 w594] -> w552
              tunnel: w550 -> [_ _]
              tunnel: w549 -> [w566 w595]
              tunnel: [w565 w595] -> w548
              tunnel: [w564 w592] -> w546
              tunnel: w547 -> [w564 w592]
              tunnel: w545 -> [w558 _]
              tunnel: w544 -> [w563 _]
              frame False {
                n189 = Strip Path(path=w558) -> (name=w562:string)  [unwired: 1 out]
                n190 = Match Pattern(string=w562, regular expression=".[Vv][Ii]$") -> (offset past match=w560:i32)  [unwired: 1 in, 3 out]
                n191 = Path To String(path=w558) -> (string=w557:string)
                n192 = case shown="0, Default" w560 {
                  tunnel: w558 -> [w588 w591]
                  tunnel: [w589 w590] -> w559
                  tunnel: [w586 _] -> w556
                  frame 0, Default {
                    n193 = Build Array(w588) -> (w587:path[])
                    n194 = call "Get VI Hierarchy Lists.vi"("Top-level VI Paths"=w587) -> ("List of VIs"=w589:path[], "error out"=w586:errorcluster)  [unwired: 11 in, 2 out]
                  }
                  frame -1 {
                    n195 = Build Array(w591) -> (w590:path[])
                  }
                }
                n196 = case shown="No Error" w556 {
                  tunnel: w566 -> [w580 w585]
                  tunnel: [w579 w584] -> w565
                  tunnel: w563 -> [w578 _]
                  tunnel: w559 -> [w574 _]
                  tunnel: w557 -> [w572 w583]
                  frame No Error {
                    n197 = Array Size(array=w574) -> (size(s)=w573:i32)
                    n198 = Build Array (concatenate)(w578, w574) -> (w577:path[])
                    n199 = Format Into String(format string="Added Hierarchy %s\nAdded %d File: " ("Message"), w572, w573) -> (resulting string=w575:string)  [unwired: 2 in, 1 out]
                    n200 = Bundle By Name(cluster=w580, "Prev File List"=w578, "File List"=w577, "Message"=w575) -> (w579:T1)
                  }
                  frame Error {
                    n201 = Concatenate Strings("Error in Adding Vi Hierarchy :" ("Message"), w583) -> (w581:string)
                    n202 = Bundle By Name(cluster=w585, "Message"=w581) -> (w584:T1)
                  }
                }
                n203 = call-poly "VIE.Module.Queued Message Handler.enqueue.State.QueuedMessageHandler.vi"("error in (no error)"=w570, "States to Enqueue"=string[] ["DisplayMessage", "DisplayFile"], "QueuedMessageHandler.dqGOOPClass (in)"=w568) -> ("error out"=w569:errorcluster, "QueuedMessageHandler.dqGOOPClass (out)"=w567:T2)  [unwired: 7 in]
              }
              frame True {
              }
            }
          }
          frame "Delete Package Integrity File" {
            n204 = Unbundle By Name(w606) -> ("Pkg File List"=w597:path[], "Package Integrity Files"=w596:i32)
            n205 = Delete From Array(array=w597, index=w596) -> (deleted portion=w599:path, array with subset deleted=w598:path[])  [unwired: 1 in]
            n206 = Path To String(path=w599) -> (string=w602:string)
            n207 = Concatenate Strings("Deleted Package Integrity File: " ("Message"), w602) -> (w600:string)
            n208 = call-poly "VIE.Module.Queued Message Handler.enqueue.State.QueuedMessageHandler.vi"("error in (no error)"=w610, "States to Enqueue"=string[] ["DisplayMessage", "DisplayPackageFile"], "QueuedMessageHandler.dqGOOPClass (in)"=w608) -> ("error out"=w609:errorcluster, "QueuedMessageHandler.dqGOOPClass (out)"=w607:T2)  [unwired: 7 in]
            n209 = Bundle By Name(cluster=w606, "Prev Pkg File List"=w597, "Pkg File List"=w598, "Message"=w600) -> (w605:T1)
          }
          frame "Remove Selected Files" {
            n210 = Unbundle By Name(w621) -> ("File List"=w616:path[], "Selected Files"=w612:i32[])
            n211 = Reverse 1D Array(array=w612) -> (reversed array=w614:i32[])
            n212 = for {
              tunnel: w614 -> [w626] mode=indexing
              shift-right: [w628] -> w617
              shift-left: w616 -> [w627]
              n213 = Delete From Array(array=w627, index=w626) -> (array with subset deleted=w628:path[])  [unwired: 1 in, 1 out]
            }
            n214 = Array Size(array=w612) -> (size(s)=w611:i32)
            n215 = Format Into String(format string="Deleted  %d Files" ("Message"), w611) -> (resulting string=w613:string)  [unwired: 2 in, 1 out]
            n216 = Bundle By Name(cluster=w621, "Prev File List"=w616, "File List"=w617, "Message"=w613) -> (w620:T1)
            n217 = call-poly "VIE.Module.Queued Message Handler.enqueue.State.QueuedMessageHandler.vi"("error in (no error)"=w625, "States to Enqueue"=string[] ["DisplayMessage", "DisplayFile"], "QueuedMessageHandler.dqGOOPClass (in)"=w623) -> ("error out"=w624:errorcluster, "QueuedMessageHandler.dqGOOPClass (out)"=w622:T2)  [unwired: 7 in]
          }
          frame "DisplayFile" {
            # "Message Queue"
            # "Message Queue"
            # "Original List"
            n218 = Unbundle By Name(w639) -> ("File List"=w642:path[], "Exclude Path"=w644:path[], "Package Integrity File Path"=w643:path)
            n219 = call-poly "Remove Duplicates from 1D Array__ogtk.vi"("Input Array"=w642) -> ("Output Array"=w653:path[])  [unwired: 1 out]
            n220 = Sort 1D Array(array=w653) -> (sorted array=w640:path[])
            n221 = for {
              tunnel: w640 -> [w663] mode=indexing
              tunnel: w644 -> [w662]
              tunnel: [w660] -> w641 mode=indexing
              n222 = call "In Any Exclude Path.vi"("Exclude Paths"=w662, "VI Path"=w663) -> ("In Any Exclude Path?"=w661:bool)  [unwired: 9 in]
              n223 = Not(x=w661) -> (.not. x?=w660:bool)
            }
            n224 = Strip Path(path=w643) -> (stripped path=w645:path)  [unwired: 1 out]
            n225 = Array Size(array=w642) -> (size(s)=w651:i32)
            n226 = Array Size(array=w640) -> (size(s)=w650:i32)
            n227 = Not Equal?(x=w651, y=w650) -> (x != y?=w652:bool)
            n228 = call "Select Element from Array.vi"("Data In"=w640, "Select?"=w641) -> ("Data Out"=w637:path[])  [unwired: 13 in]
            n229 = case shown="True" w652 {
              tunnel: w651 -> [_ w671]
              tunnel: w650 -> [_ w672]
              tunnel: [_ w668] -> w631
              frame False {
              }
              frame True {
                n230 = Subtract(x=w671, y=w672) -> (x-y=w669:i32)
                n231 = Format Into String(format string="    %d Repeated File(s) Found and Removed from List" ("Format String"), w669) -> (resulting string=w668:string)  [unwired: 2 in, 1 out]
              }
            }
            n232 = Array Size(array=w640) -> (size(s)=w648:i32)
            n233 = Array Size(array=w637) -> (size(s)=w647:i32)
            n234 = for {
              tunnel: w645 -> [w667]
              tunnel: w637 -> [w666] mode=indexing
              tunnel: [w664] -> w649 mode=indexing
              n235 = call "Abs to Rel Path.vi"("File Path"=w666, "Base Path"=w667) -> ("Path Out"=w665:path)  [unwired: 8 in, 1 out]
              n236 = Path To String(path=w665) -> (string=w664:string)
            }
            n237 = Not Equal?(x=w648, y=w647) -> (x != y?=w646:bool)
            n238 = case shown="True" w646 {
              tunnel: w648 -> [_ w658]
              tunnel: w647 -> [_ w659]
              tunnel: [_ w655] -> w630
              frame False {
              }
              frame True {
                n239 = Subtract(x=w658, y=w659) -> (x-y=w656:i32)
                n240 = Format Into String(format string="    %d File(s) In Exclude Paths, therefore Removed" ("Format String"), w656) -> (resulting string=w655:string)  [unwired: 2 in, 1 out]
              }
            }
            n241 = call-poly "VIE.Module.Queued Message Handler.enqueue.State.QueuedMessageHandler.vi"("error in (no error)"=w635, "States to Enqueue"=string[] ["DisplayMessage", "DisplayPackageFile"], "QueuedMessageHandler.dqGOOPClass (in)"=w633) -> ("error out"=w634:errorcluster, "QueuedMessageHandler.dqGOOPClass (out)"=w632:T2)  [unwired: 7 in]
            n242 = property on="File List" class="LstBox (strict)"("Item Names"=w649) -> ()  [unwired: 2 in, 2 out]
            n243 = Concatenate Strings(w630, w631) -> (w629:string)
            n244 = Bundle By Name(cluster=w639, "File List"=w637, "Message"=w629) -> (w638:T1)
          }
          frame "---- System States --------------------------" {
            # "Do not put any code in here - this is a case divider, and is not a valid state, so any code here will not be executed."
          }
          frame "system.StateNameSyntaxError", Default {
            # "Do not alter the code in here - this is a system state that is required by the state machine architecture."
            n245 = property class="VI"() -> ("Name"=w682:string)  [unwired: 2 in, 2 out]
            n246 = Format Into String(format string="Syntax Error - Requested State not found in State Machine Architecture.\n\nArchitecture: %s\nState Requested: %s", w682, w679) -> (resulting string=w683:string)  [unwired: 2 in, 1 out]
            n247 = call <vilib>:"Error Cluster From Error Code.vi"("error in (no error)"=w681, "error message (\"\")"=w683, "error code (0)"=46) -> ("error out"=w680:errorcluster)  [unwired: 6 in]
          }
          frame "system.HandleErrors" {
            # "Do not alter the code in here - this is a system state that is required by the state machine architecture."
            # "Handle errors by presenting a dialog box to the\nuser and logging the error to file (if enabled)"
            n248 = call <vilib>:"Simple Error Handler.vi"("error in (no error)"=w698) -> ("code out"=w694:i32, "source out"=w693:string, "error out"=w695:errorcluster)  [unwired: 4 in, 2 out]
            n249 = Format Into String(format string="ERROR: Code=%d, Source=\"%s\"", w694, w693) -> (resulting string=w692:string)  [unwired: 2 in, 1 out]
            n250 = call <vilib>:"Clear Errors.vi"("error in (no error)"=w695) -> ("error out"=w691:errorcluster)  [unwired: 6 in]
            n251 = call "VIE.Module.Queued Message Handler.logEvent.QueuedMessageHandler.vi"("error in (no error)"=w696, "Event to Log"=w692, "QueuedMessageHandler.dqGOOPClass (in)"=w697) -> ("error out"=w689:errorcluster, "QueuedMessageHandler.dqGOOPClass (out)"=w690:T2)  [unwired: 7 in]
            n252 = disable-structure shown="Enabled" {
              disable-tunnel: w690 -> [w705 w710 w711]
              disable-tunnel: w689 -> [w704 w709 w712]
              disable-tunnel: [w703 w708 w711] -> w688
              disable-tunnel: [w702 w707 w712] -> w687
              frame Disabled {
                # "Enable this case to force software\nto exit on error."
                n253 = call-poly "VIE.Module.Queued Message Handler.enqueue.State.QueuedMessageHandler.vi"("error in (no error)"=w704, "State to Enqueue"="system.Exit", "QueuedMessageHandler.dqGOOPClass (in)"=w705) -> ("error out"=w702:errorcluster, "QueuedMessageHandler.dqGOOPClass (out)"=w703:T2)  [unwired: 7 in]
              }
              frame Disabled {
                # "Enable this case to force software\nto cleanup then exit on error."
                n254 = call-poly "VIE.Module.Queued Message Handler.enqueue.State.QueuedMessageHandler.vi"("error in (no error)"=w709, "States to Enqueue"=string[] ["custom.CleanUp", "system.Exit"], "QueuedMessageHandler.dqGOOPClass (in)"=w710) -> ("error out"=w707:errorcluster, "QueuedMessageHandler.dqGOOPClass (out)"=w708:T2)  [unwired: 7 in]
              }
              frame Enabled {
                # "Enable this case to force software\nto continue on error."
              }
            }
          }
          frame "system.Exit" {
            # "Enable this case to leave all local data added in this VI in the CVT to be\npassed out to the calling VI"
            # "Do not alter the code in here - this is a system state that is required by the state machine architecture."
          }
        }
        n255 = case shown="Error" w26 {
          tunnel: w25 -> [w35 w41]
          tunnel: w24 -> [w36 w40]
          tunnel: [w35 w39] -> w23
          tunnel: [w36 w38] -> w22
          frame No Error {
          }
          frame Error {
            n256 = call "VIE.Module.Queued Message Handler.flush.QueuedMessageHandler.vi"("error in (no error)"=w41, "QueuedMessageHandler.dqGOOPClass (in)"=w40) -> ("error out"=w43:errorcluster, "QueuedMessageHandler.dqGOOPClass (out)"=w42:T2)  [unwired: 7 in, 1 out]
            n257 = call-poly "VIE.Module.Queued Message Handler.enqueue.State.QueuedMessageHandler.vi"("error in (no error)"=w43, "State to Enqueue"="system.HandleErrors", "QueuedMessageHandler.dqGOOPClass (in)"=w42) -> ("error out"=w39:errorcluster, "QueuedMessageHandler.dqGOOPClass (out)"=w38:T2)  [unwired: 7 in]
          }
        }
      }
      n258 = call "VIE.Module.Queued Message Handler.destroy.QueuedMessageHandler.vi"("error in (no error)"=w14, "QueuedMessageHandler.dqGOOPClass (in)"=w13) -> ()  [unwired: 9 in, 1 out]
    }
    frame Error {
      # "An error was passed into the VI, so do not execute and pass the error and input CVT out."
    }
  }
  "error out" <- w2
  "CVT (out)" <- w4
